vi "Stop.vi"(8 "error in (no error)":errorcluster, 11 "UI in":refnum<class "UI.lvclass">) -> (0 "error out":errorcluster, 3 "UI out":refnum<class "UI.lvclass">)   [LabVIEW 2018]
uses:
  UI/UI.lvclass
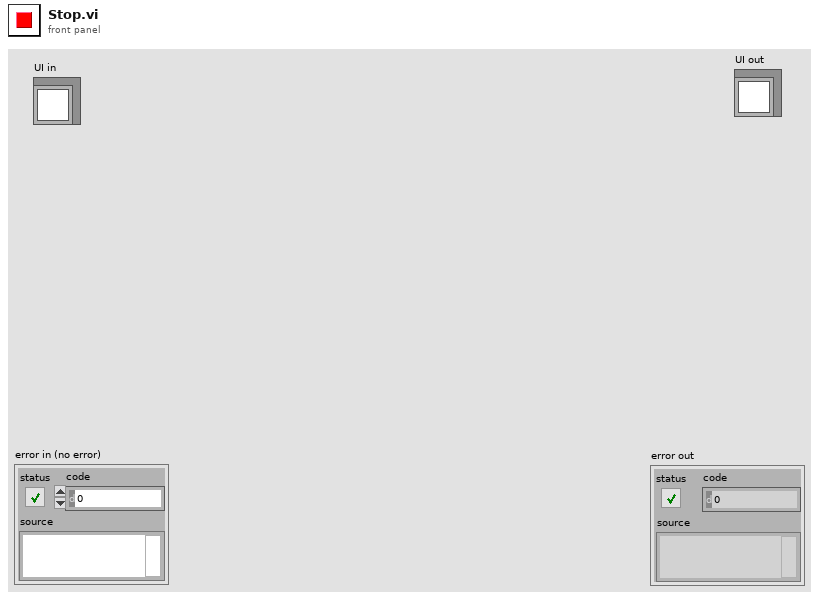
[diagram p1: front panel]
types:
  T1 = enum16{"Create", "Register", "Generate", "Unregister", "Destroy"}
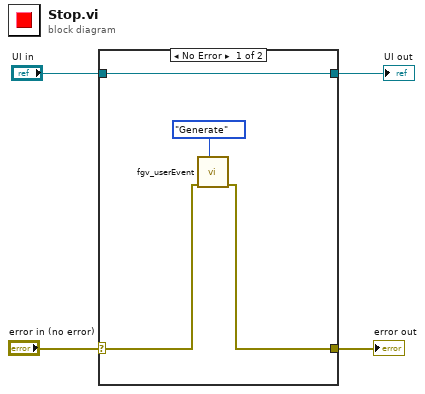
[diagram p0: block diagram]
diagram:
  n1 = case shown="No Error" "error in (no error)" {
    selector: "error in (no error)" -> [w7 w9]
    tunnel: [w6 w9] -> w3
    tunnel: "UI in" -> [w5 w10]
    tunnel: [w5 w10] -> w1
    frame No Error {
      n2 = call "fgv_userEvent.vi"("Option"=T1."Generate", "Error In"=w7) -> ("Error Out"=w6:errorcluster)  [unwired: 8 in, 1 out]
    }
    frame Error {
    }
  }
  "UI out" <- w1
  "error out" <- w3
